vi "Random Number In Range.vi"(1 "Lower Limit":u32, 2 "Upper Limit":u32=1) -> (0 "Random #":u32)   [LabVIEW 2016]
doc: "Returns a random number in the range specified by the upper and lowe limits."
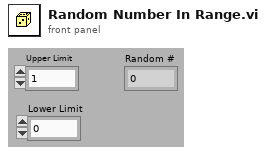
[diagram p1: front panel]
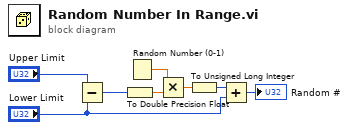
[diagram p0: block diagram]
diagram:
  n1 = Subtract(x="Upper Limit", y="Lower Limit") -> (x-y=w6:u32)
  n2 = To Double Precision Float(number=w6) -> (double precision float=w2:dbl)
  n3 = Random Number (0-1)() -> (number: 0 to 1=w3:dbl)
  n4 = Multiply(x=w3, y=w2) -> (x*y=w8:dbl)
  n5 = To Unsigned Long Integer(number=w8) -> (unsigned 32bit integer=w1:u32)
  n6 = Add(x=w1, y="Lower Limit") -> (x+y=→"Random #":u32)
